vi "Ref info.vi"(8 "error in (no error)":errorcluster, 11 "Variant":variant) -> (0 "error out":errorcluster, 2 "refnum type":variant, 3 "child strings":string[](array[string]))   [LabVIEW 2017, in "DSF Configuration Utility.lvlib"]
uses:
  DSF Configuration Utility.lvlib
  <vilib>/Utility/Data Type/NI_Data Type.lvlib
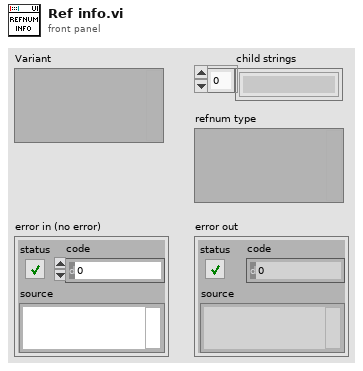
[diagram p1: front panel]
types:
  T1 = typedef "NI_Data Type.lvlib/VI Server Generic Type.ctl" = enum16{"NoType", "\tkLVObjApp=0x1", "\tkLVObjVI", "\tkLVObjGeneric", "\tkLVObjDecoration", "\tkLVObjText", "\tkLVObjControl", "\tkLVObjColorBox", "\tkLVObjBoolean", "\tkLVObjRefNum", "\tkLVObjVariant", "\tkLVObjPath", "\tkLVObjListBox", "\tkLVObjTable", "\tkLVObjArray", "\tkLVObjPicture", "\tkLVObjOleContainer", "\tkLVObjNumeric", "\tkLVObjDigital", "\tkLVObjNamedNumeric", "\tkLVObjColorRamp", "\tkLVObjSlide", "\tkLVObjGraphOrChart", "\tkLVObjWaveformChart", "\tkLVObjWaveformGraph", "\tkLVObjIntensityChart", "\tkLVObjIntensityGraph", "\tkLVObjString", "\tkLVObjIOName", "\tkLVObjComboBox", "\tkLVObjCluster", "\tkLVObjPanel", "\tkLVObjKnob", "\tkLVObjNumWithScale", "\tkLVObjRing", "\tkLVObjEnum", "\tkLVObjGObject", "\tkLVObjPlot", "\tkLVObjCursor", "\tkLVObjNumericText", "\tkLVObjScale", "\tkLVObjColorScale", "\tkLVObjGraphScale", "\tkLVObjColorGraphScale", "\tkLVObjTypedRefNum", "\tkLVObjOldKnobScale", "\tkLVObjMCListbox", "\tkLVObjMeasureData", "\tkLVObjDSCTag", "\tkLVObjDAQName", "\tkLVObjVISAName", "\tkLVObjIVIName", "\tkLVObjSlideScale", "\tkLVObjTabControl", "\tkLVObjPage", "\tkLVObjTabArrayTabControl", "\tkLVObjConPane", "\tkLVObjDAQMXName", "\tkLVObjVIRefNum", "\tkLVObjLVObjRefNum", "\tkLVObjAbsTime", "\tkLVObjDigitalTable", "\tkLVObjUnused", "\tkLVObjUnused2", "\tkLVObjSCLControl", "\tkLVObjSubPanel", "\tkLVObjTreeControl", "\tkLVObjGenClassTagRef", "\tkLVObjGenClassRef", "\tkLVObjRotaryColorScale", "\tkLVObjPlugInDDOControl", "\tkLVObjPlugInDDOClassHolder", "\tkLVObjRadClusControl", "\tkLVObjProject", "\tkLVObjProjectItem", "\tkLVObjPane", "\tkLVObjSplitterBar", "\tkLVObjProjectBuildItem", "\tkLVObjPixmap", "\tkLVObjFacadeVI", "\tkLVObjLibrary", "\tkLVObjVariable", "\tkLVObjPropertyBag", "\tkLVObjXYGraph", "\tkLVObjScene", "\tkLVObjUDClassLibrary", "\tkLVObjUDClassClone", "\tkLVObjMethodVI", "\tkLVObjXCtlLibrary", "\tkLVObjXNodeLibrary", "\tkLVObjScroll", "\tkLVObjLVTarget", "\tkLVObjMixedGraph", "\tkLVObjProvider", "\tkLVObjCopyOperation", "\tkLVObjTargetItem", "\tkLVObjProjectItemType", "\tkLVObjCopyItem", "\tkLVObjCopyConflict", "\tkLVObjCopyExpert", "\tkLVObjSceneGraphDisp", "\tkLVObjPolyVI", "\tkLVObjLVClassDDO", "kLVObjDiagram=0x4000", "\tkLVObjTerminal", "\tkLVObjConstant", "\tkLVObjPathConstant", "\tkLVObjArrayConstant", "\tkLVObjNumericConstant", "\tkLVObjDigitalNumConstant", "\tkLVObjNamedNumericConstant", "\tkLVObjStringConstant", "\tkLVObjClusterConstant", "\tkLVObjFixedConstant", "\tkLVObjControlTerminal", "\tkLVObjFormulaParameter", "\tkLVObjGlobal", "\tkLVObjLocal", "\tkLVObjRightShiftRegister", "\tkLVObjFunction", "\tkLVObjSubVI", "\tkLVObjCallByRef", "\tkLVObjUnitCast", "\tkLVObjStructure", "\tkLVObjLoop", "\tkLVObjMultiframeStructure", "\tkLVObjSequence", "\tkLVObjCaseSelector", "\tkLVObjFormula", "\tkLVObjGrowableFunction", "\tkLVObjBuildClusterArray", "\tkLVObjCompoundArithmetic", "\tkLVObjIndexArray", "\tkLVObjBuildArray", "\tkLVObjNamedBundler", "\tkLVObjCIN", "\tkLVObjCallLibrary", "\tkLVObjObjectFunction", "\tkLVObjProperty", "\tkLVObjInvoke", "\tkLVObjNode", "\tkLVObjBooleanConstant", "\tkLVObjBlockDiagram", "\tkLVObjRingConstant", "\tkLVObjEnumConstant", "\tkLVObjTunnel", "\tkLVObjLoopTunnel", "\tkLVObjSequenceLocal", "\tkLVObjComparison", "\tkLVObjReadWriteFile", "\tkLVObjTypeCast", "\tkLVObjFlattenUnflattenString", "\tkLVObjGPIBReadWrite", "\tkLVObjForLoop", "\tkLVObjWhileLoop", "\tkLVObjScriptNode", "\tkLVObjArrayToCluster", "\tkLVObjFormatScanString", "\tkLVObjWire", "\tkLVObjProbe", "\tkLVObjInnerTerminal", "\tkLVObjLeftShiftRegister", "\tkLVObjPolySubVI", "\tkLVObjPropItem", "\tkLVObjIONameConstant", "\tkLVObjDSCTagConstant", "\tkLVObjDAQNameConstant", "\tkLVObjVISANameConstant", "\tkLVObjIVINameConstant", "\tkLVObjColorBoxConstant", "\tkLVObjControlRefConstant", "\tkLVObjClassSpecifierConstant", "\tkLVObjConfNode", "\tkLVObjMasterWizard", "\tkLVObjStateDiagWizard", "\tkLVObjOuterTerminal", "\tkLVObjDAQMXNameConstant", "\tkLVObjEventStructure", "\tkLVObjFlatSequence", "\tkLVObjGenClassTagRefConstant", "\tkLVObjAbsTimeConstant", "\tkLVObjExternalNode", "\tkLVObjSubWizard", "\tkLVObjScriptNodeParameter", "\tkLVObjStatVIRef", "\tkLVObjComboBoxConstant", "\tkLVObjTimedLoop", "\tkLVObjGenClassDeepCopy", "\tkLVObjGenClassTagFlat", "\tkLVObjGenClassTagFlatRefConstant", "\tkLVObjGenClassFlat", "\tkLVObjSimDiagram", "\tkLVObjCompDiagram", "\tkLVObjSimNode", "\tkLVObjSimDCO", "\tkLVObjBundler", "\tkLVObjUnbundler", "\tkLVObjNamedUnbundler", "\tkLVObjFlatSeqFrame", "\tkLVObjFlatSeqInTun", "\tkLVObjFlatSeqOutTun", "\tkLVObjRefNumConst", "\tkLVObjFlattenString", "\tkLVObjPolySelector", "\tkLVObjXNode", "\tkLVObjSelectorTunnel", "\tkLVObjCommentNode", "\tkLVObjSdfDiagram", "\tkLVObjSDFCompDiagram", "\tkLVObjSdfNode", "\tkLVObjSdfDCO", "\tkLVObjFileDialog", "\tkLVObjTLDCO", "\tkLVObjTimeSeqFrame", "\tkLVObjTimeFlatSequence", "\tkLVObjTimedSequence", "\tkLVObjXDataNode", "\tkLVObjCodeWizard", "\tkLVObjMathScriptNode", "\tkLVObjMathScriptNodeParameter", "\tkLVObjLVClassBDConst"}
  T2 = typedef "NI_Data Type.lvlib/Refnum Type.ctl" = enum16{"NotARefnum", "UnknownRefnum", "Generic", "Datalog", "ByteStream", "Device", "Occurence", "TCPNetConnection", "Auto", "Menu", "Imaq", "Hardware", "DataSocket", "Visa", "IVI", "UDPNetConnection", "Notifier", "Queue", "Irda", "EventReg", "DotNet", "UserEvent", "Callback", "UNUSED_EMPTY_POSITION", "BlueToothNetConnection", "LVObjApp", "LVObjVI", "LVObjUnknown", "GenericClass", "UserDefinedRefnumTag", "DataValue", "RT FIFO", "TDMS File"}
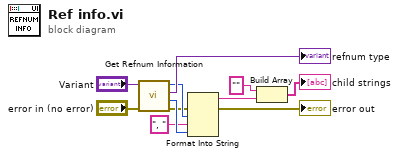
[diagram p0: block diagram]
diagram:
  n1 = call <vilib>:"Get Refnum Information.vi"("error in (no error)"="error in (no error)", "Variant"="Variant") -> ("error out"=w3:errorcluster, "VI Server Generic Type"=w8:T1, "Strict Type"=→"refnum type":variant, "Reference Type"=w6:T2)  [unwired: 6 in]
  n2 = Format Into String(error in=w3, w6, ", ", w8) -> (resulting string=w9:string, error out=→"error out":errorcluster)  [unwired: 2 in]
  n3 = Build Array("" ("element"), w9) -> (→"child strings":string[])
